vi "Add Remove Culled Object.vi"(7 "SensorInfo":T1={"Sensor Name"="", "Protocol"=enum."UDP", "Network port"=48185, "# Culled Objects"=1, "PlayerID"=1, "MM Data"=[]}, 8 "error in (no error)":errorcluster, 11 "Item Ref in":T7 format="%.0x") -> (0 "error out (no error)":errorcluster)   [LabVIEW 2023, in "Vires VTD System Explorer.lvlib"]
uses:
  Vires VTD System Explorer.lvlib
  <vilib>/NI VeriStand/Custom Device API/Custom Device Item Ref.ctl
  Shared/SensorInfo.ctl
  Shared/Sensor Name.ctl
  Shared/Protocol.ctl
  MM/MM Data.ctl
  MM/MM Objects.ctl
  MM/MM Object.ctl
  <vilib>/NI VeriStand/Custom Device API/Custom Device Channel.ctl
  <vilib>/NI VeriStand/Custom Device API/Custom Device Channel Type.ctl
  Shared/Constants.vi
  <vilib>/NI VeriStand/Custom Device API/Set Item Property (Variant).vi
  <vilib>/NI VeriStand/Custom Device API/Custom Device API.lvlib
  Shared/Vires VTD Shared.lvlib
  MM/MM.lvlib
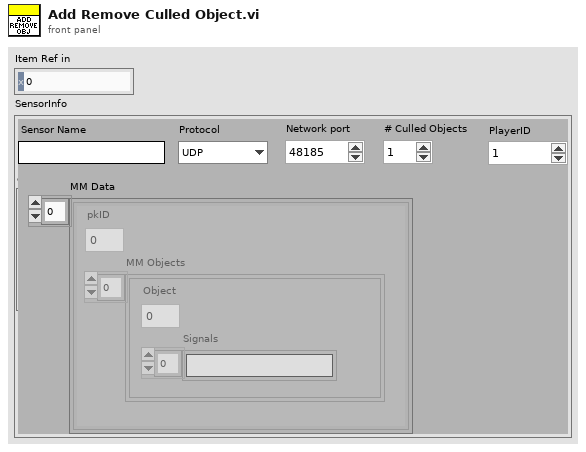
[diagram p1: front panel]
types:
  T1 = typedef "Vires VTD Shared.lvlib/SensorInfo.ctl" = cluster{"Sensor Name":T2, "Protocol":T3, "Network port":i32, "# Culled Objects":i32, "PlayerID":u8, "MM Data":T4}
  T2 = typedef "Vires VTD Shared.lvlib/Sensor Name.ctl" = string
  T3 = typedef "Vires VTD Shared.lvlib/Protocol.ctl" = enum16{"UDP", "TCP"}
  T4 = typedef "Vires VTD Shared.lvlib/MM Data.ctl" = T5[]
  T5 = typedef "MM.lvlib/MM Objects.ctl" = cluster{"pkID":i32, "MM Objects":T6[]}
  T6 = typedef "MM.lvlib/MM Object.ctl" = cluster{"Object":i32, "Signals":string[]}
  T7 = typedef "Custom Device API.lvlib/Custom Device Item Ref.ctl" = u64
  T8 = typedef "Custom Device API.lvlib/Custom Device Channel.ctl" = cluster{"Type":T9, "Units":string, "Default Value":dbl, "Faultable":bool, "Scalable":bool}
  T9 = typedef "Custom Device API.lvlib/Custom Device Channel Type.ctl" = enum16{"Input", "Output"}
  T10 = typedef "Custom Device API.lvlib/Custom Device Item Info.ctl" = cluster{"Name":string, "Is Channel":bool, "GUID":string, "Is Waveform":bool}
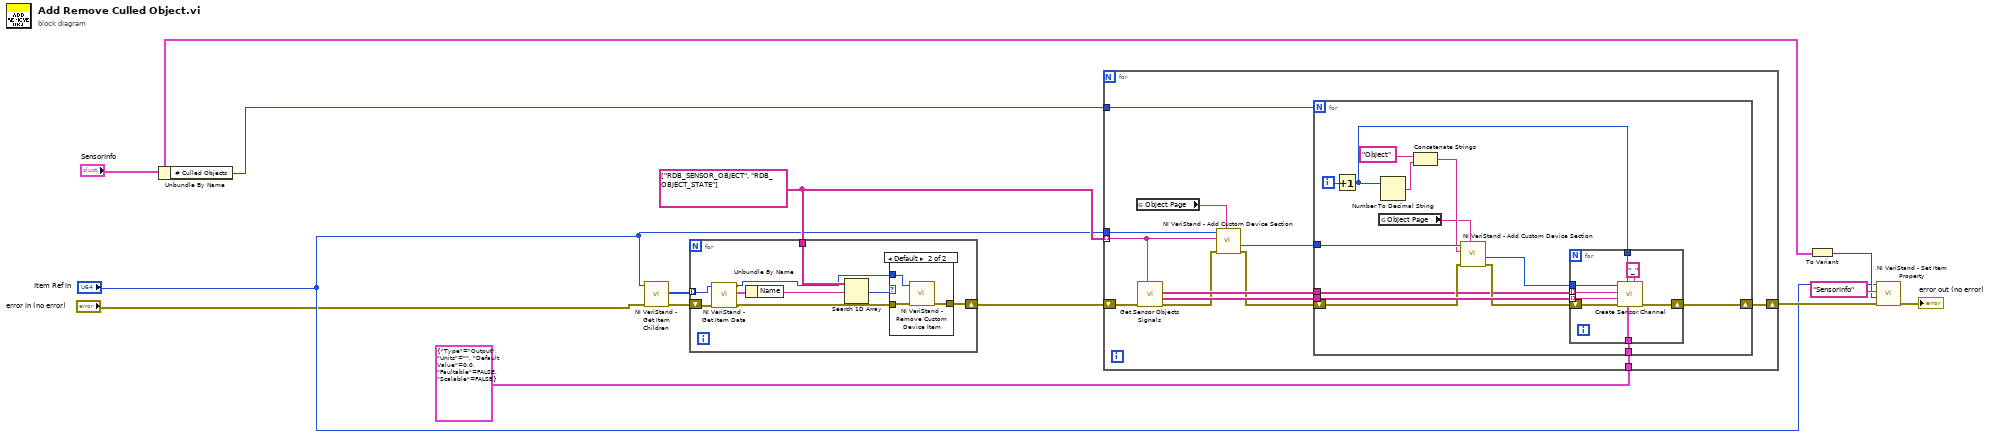
[diagram p0: block diagram]
diagram:
  w4 = string[] ["RDB_SENSOR_OBJECT", "RDB_OBJECT_STATE"]
  n1 = Unbundle By Name("SensorInfo") -> ("# Culled Objects"=w13:i32)
  n2 = call <vilib>:"NI VeriStand - Get Item Children.vi"("error in (no error)"="error in (no error)", "Item Ref in"="Item Ref in") -> ("error out"=w5:errorcluster, "Child Refs"=w6:T7[])  [unwired: 6 in, 2 out]
  n3 = for {
    tunnel: w6 -> [w16] mode=indexing
    shift-right: [w20] -> w3
    shift-left: w5 -> [w18]
    tunnel: w4 -> [w22]
    n4 = call <vilib>:"NI VeriStand - Get Item Data.vi"("error in (no error)"=w18, "Item Ref in"=w16) -> ("error out"=w17:errorcluster, "Item Info"=w19:T10, "Item Ref out"=w14:T7)  [unwired: 7 out]
    n5 = Unbundle By Name(w19) -> ("Name"=w15:string)
    n6 = Search 1D Array(1D array=w22, element=w15) -> (index of element=w21:i32)  [unwired: 1 in]
    n7 = case shown="Default" w21 {
      tunnel: w17 -> [w23 w26]
      tunnel: [w23 w25] -> w20
      tunnel: w14 -> [_ w24]
      frame -1 {
      }
      frame Default {
        n8 = call <vilib>:"NI VeriStand - Remove Custom Device Item.vi"("error in (no error)"=w26, "Item Ref in"=w24) -> ("error out"=w25:errorcluster)  [unwired: 8 in, 1 out]
      }
    }
  }
  n9 = for {
    tunnel: w13 -> [w36]
    tunnel: T8 {"Type"=enum."Output", "Units"="", "Default Value"=0.0, "Faultable"=FALSE, "Scalable"=FALSE} ("Channel") -> [w35]
    tunnel: "Item Ref in" -> [w32]
    shift-right: [w37] -> w11
    shift-left: w3 -> [w38]
    tunnel: w4 -> [w29] mode=indexing
    n10 = global read "Constants.vi" "Object Page"() -> (w28:string)
    n11 = call "Get Sensor Objects Signals.vi"("Filter Cluster"=w29, "error in (no error)"=w38) -> ("error out (no error)"=w31:errorcluster, "Sensor Signals"=w34:string[], "Sensor Names"=w33:string[])  [unwired: 7 in]
    n12 = call <vilib>:"NI VeriStand - Add Custom Device Section.vi"("GUID (Default Section)"=w28, "error in (no error)"=w31, "Section Name"=w29, "Parent Ref in"=w32) -> ("error out"=w30:errorcluster, "Section Ptr"=w27:T7)  [unwired: 4 in, 2 out]
    n13 = for {
      N: w36 -> [_]
      shift-right: [w52] -> w37
      shift-left: w30 -> [w49]
      tunnel: w35 -> [w51]
      tunnel: w34 -> [w50]
      tunnel: w27 -> [w47]
      tunnel: w33 -> [w40]
      i -> [w44]
      n14 = Increment(x=w44) -> (x+1=w39:i32)
      n15 = global read "Constants.vi" "Object Page"() -> (w41:string)
      n16 = Number To Decimal String(number=w39) -> (decimal integer string=w43:string)  [unwired: 1 in]
      n17 = Concatenate Strings("Object" ("Section Name"), w43) -> (w42:string)
      n18 = call <vilib>:"NI VeriStand - Add Custom Device Section.vi"("GUID (Default Section)"=w41, "error in (no error)"=w49, "Section Name"=w42, "Parent Ref in"=w47) -> ("error out"=w48:errorcluster, "Section Ptr"=w46:T7)  [unwired: 4 in, 2 out]
      n19 = for {
        tunnel: w51 -> [w54]
        shift-right: [w60] -> w52
        shift-left: w48 -> [w59]
        tunnel: w46 -> [w58]
        tunnel: w39 -> [w57]
        tunnel: w50 -> [w53] mode=indexing
        tunnel: w40 -> [w56] mode=indexing
        n20 = call "Create Sensor Channel.vi"("regular expression"="_", "Channel"=w54, "Object"=w57, "error in (no error)"=w59, "RDB Signalname"=w53, "RDB Receive Objects"=w56, "Item Ref in"=w58) -> ("error out"=w60:errorcluster)  [unwired: 3 in, 1 out]
      }
    }
  }
  n21 = To Variant(anything="SensorInfo") -> (Variant=w8:variant)
  n22 = call-poly <vilib>:"NI VeriStand - Set Item Property.vi"("error in (no error)"=w11, "Value"=w8, "Property Name"="SensorInfo" ("String"), "Item Ref in"="Item Ref in") -> ("error out"=→"error out (no error)":errorcluster)  [unwired: 5 in, 2 out]
